vi "Script Error.vi"(0 "Error?":bool, 1 "Reset Log":bool, 2 "Error Details":string, 3 "Error Code":i32, 4 "Line Number":i32) -> (5 "Error?":bool)   [LabVIEW 2017, in "Apple script.lvlib"]
uses:
  Apple script.lvlib
  <vilib>/Rock Robotics/Network Tables/NT Write String.vi
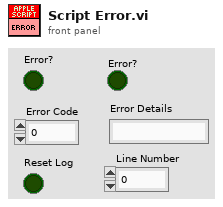
[diagram p1: front panel]
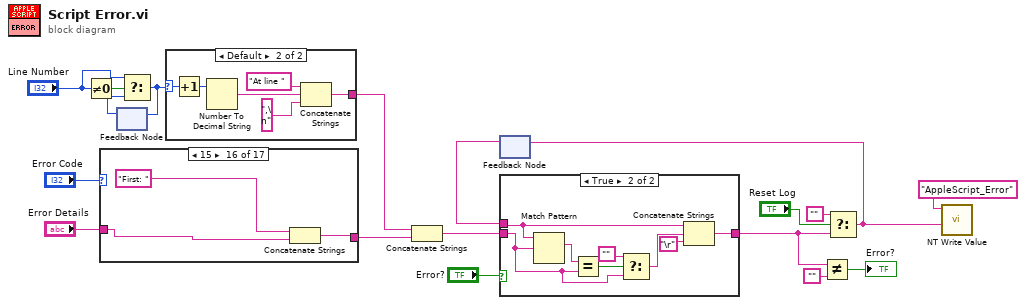
[diagram p0: block diagram]
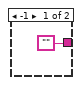
[diagram p2: hidden frame]
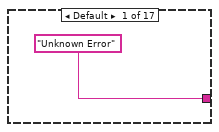
[diagram p4: hidden frame]
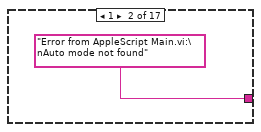
[diagram p5: hidden frame]
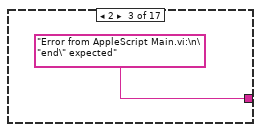
[diagram p6: hidden frame]
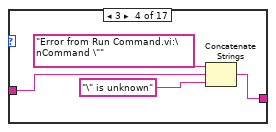
[diagram p7: hidden frame]
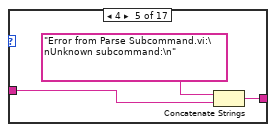
[diagram p8: hidden frame]
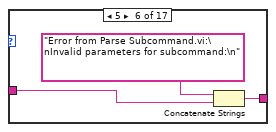
[diagram p9: hidden frame]
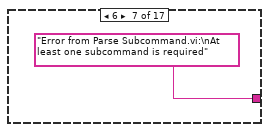
[diagram p10: hidden frame]
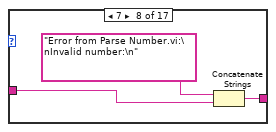
[diagram p11: hidden frame]
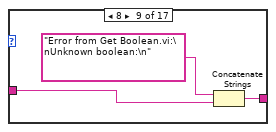
[diagram p12: hidden frame]
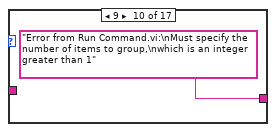
[diagram p13: hidden frame]
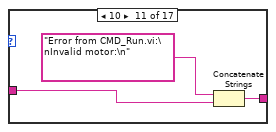
[diagram p14: hidden frame]
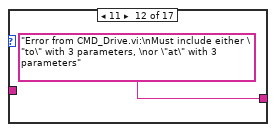
[diagram p15: hidden frame]
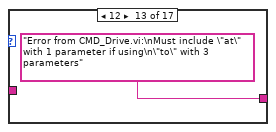
[diagram p16: hidden frame]
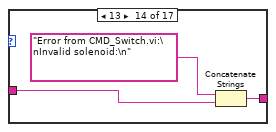
[diagram p17: hidden frame]
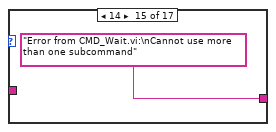
[diagram p18: hidden frame]
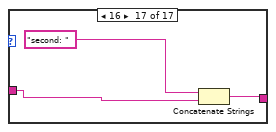
[diagram p19: hidden frame]
diagram:
  n1 = Not Equal To 0?(x="Line Number") -> (x != 0?=w9:bool)
  n2 = case shown="15" "Error Code" {
    tunnel: ["Unknown Error" "Error from AppleScript Main.vi:\nAuto mode not found" "Error from AppleScript Main.vi:\n\"end\" expected" w23 w26 w29 "Error from Parse Subcommand.vi:\nAt least one subcommand is required" w33 w36 "Error from Run Command.vi:\nMust specify the number of items to group,\nwhich is an integer greater than 1" w40 "Error from CMD_Drive.vi:\nMust include either \"to\" with 3 parameters, \nor \"at\" with 3 parameters" "Error from CMD_Drive.vi:\nMust include \"at\" with 1 parameter if using\n\"to\" with 3 parameters" w45 "Error from CMD_Wait.vi:\nCannot use more than one subcommand" w50 w53] -> w14
    tunnel: "Error Details" -> [_ _ _ w24 w27 w30 _ w34 w37 _ w41 _ _ w46 _ w49 w52]
    frame Default {
    }
    frame 1 {
    }
    frame 2 {
    }
    frame 3 {
      n3 = Concatenate Strings("Error from Run Command.vi:\nCommand \"", w24, "\" is unknown" ("string")) -> (w23:string)
    }
    frame 4 {
      n4 = Concatenate Strings("Error from Parse Subcommand.vi:\nUnknown subcommand:\n", w27) -> (w26:string)
    }
    frame 5 {
      n5 = Concatenate Strings("Error from Parse Subcommand.vi:\nInvalid parameters for subcommand:\n", w30) -> (w29:string)
    }
    frame 6 {
    }
    frame 7 {
      n6 = Concatenate Strings("Error from Parse Number.vi:\nInvalid number:\n", w34) -> (w33:string)
    }
    frame 8 {
      n7 = Concatenate Strings("Error from Get Boolean.vi:\nUnknown boolean:\n", w37) -> (w36:string)
    }
    frame 9 {
    }
    frame 10 {
      n8 = Concatenate Strings("Error from CMD_Run.vi:\nInvalid motor:\n", w41) -> (w40:string)
    }
    frame 11 {
    }
    frame 12 {
    }
    frame 13 {
      n9 = Concatenate Strings("Error from CMD_Switch.vi:\nInvalid solenoid:\n", w46) -> (w45:string)
    }
    frame 14 {
    }
    frame 15 {
      n10 = Concatenate Strings("First: ", w49) -> (w50:string)
    }
    frame 16 {
      n11 = Concatenate Strings("second: ", w52) -> (w53:string)
    }
  }
  n12 = feedback #1() -> (w8:i32)  [unwired: 1 in]
  n13 = Select(t="Line Number", s=w9, f=w8) -> (s? t:f=w7:i32)
  n14 = feedback-in #1(w7) -> ()
  n15 = case shown="Default" w7 {
    selector: w7 -> [_ w57]
    tunnel: ["" w59] -> w13
    frame -1 {
    }
    frame Default {
      n16 = Increment(x=w57) -> (x+1=w56:i32)
      n17 = Number To Decimal String(number=w56) -> (decimal integer string=w61:string)  [unwired: 1 in]
      n18 = Concatenate Strings("At line " ("string"), w61, ",\n" ("string")) -> (w59:string)
    }
  }
  n19 = Concatenate Strings(w13, w14) -> (w11:string)
  n20 = feedback #2() -> (w12:string)  [unwired: 1 in]
  n21 = case shown="True" "Error?" {
    tunnel: w11 -> [_ w66]
    tunnel: w12 -> [w62 w68]
    tunnel: [w62 w70] -> w5
    frame False {
    }
    frame True {
      n22 = Match Pattern(string=w68, regular expression=w66) -> (match substring=w69:string)  [unwired: 1 in, 3 out]
      n23 = Equal?(x=w69, y=w66) -> (x = y?=w67:bool)
      n24 = Select(t="", s=w67, f=w66) -> (s? t:f=w64:string)
      n25 = Concatenate Strings(w68, w64, "\r") -> (w70:string)
    }
  }
  n26 = Not Equal?(x=w5, y="") -> (x != y?=→"Error?":bool)
  n27 = Select(t="", s="Reset Log", f=w5) -> (s? t:f=w1:string)
  n28 = feedback-in #2(w1) -> ()
  n29 = call-poly <vilib>:"NT Write Value.vi"("String"=w1, "Name"="AppleScript_Error") -> ()  [unwired: 9 in, 1 out]
